vi "Init.vi"(8 "Error In":errorcluster, 10 "Folder Path":path, 11 "Protocol Interface in":refnum<class "Protocol Interface.lvclass">) -> (0 "Error Out":errorcluster, 3 "Protocol Interface out":refnum<class "Protocol Interface.lvclass">)   [LabVIEW 2018, in "Protocol Interface.lvlib" / "Protocol Interface.lvclass"]
uses:
  Protocol Interface.lvclass
  FPF.lvlibp/Factory Plugin Framework.lvclass
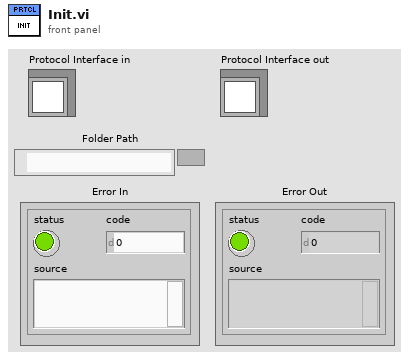
[diagram p1: front panel]
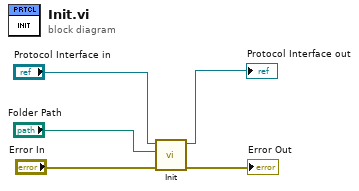
[diagram p0: block diagram]
diagram:
  n1 = call-parent "Init.vi"("Error In"="Error In", "Folder Path"="Folder Path", "Plugin Framework In"="Protocol Interface in") -> ("Error Out"=→"Error Out":errorcluster, "Factory Plugin Framework out"=→"Protocol Interface out":refnum<class "Protocol Interface.lvclass">)  [unwired: 7 in]
